vi "Determine XML Dependencies Paths.vi"(10 "Execution Mode":T1, 11 "Targets":enum16{"Linux_x64", "Windows", "All"}(ring)) -> (1 "Targets":string[](array[string]), 2 "Target Paths":string[](array[string]), 3 "Source Paths":string[](array[string]))   [LabVIEW 2026, in "NIVS_CDEW_MetaDataObj.lvclass"]
uses:
  Types/Execution Modes.ctl
  NIVS_CDEW_MetaDataObj.lvclass
  NIVS_CDEW_MetaDataObj.lvclass/NIVS_CDEW_MetaDataObj.ctl
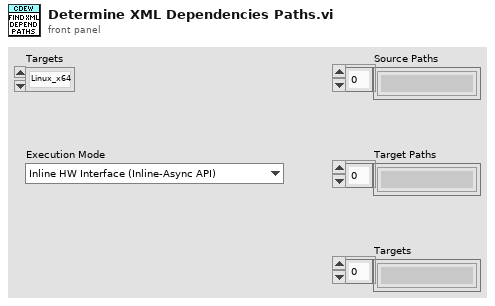
[diagram p1: front panel]
types:
  T1 = typedef "NIVS_CDEW_MetaDataObj.lvclass/Execution Modes.ctl" = enum16{"Inline HW Interface (Inline-Async API)", "Inline HW Interface", "Inline Timing and Sync"}
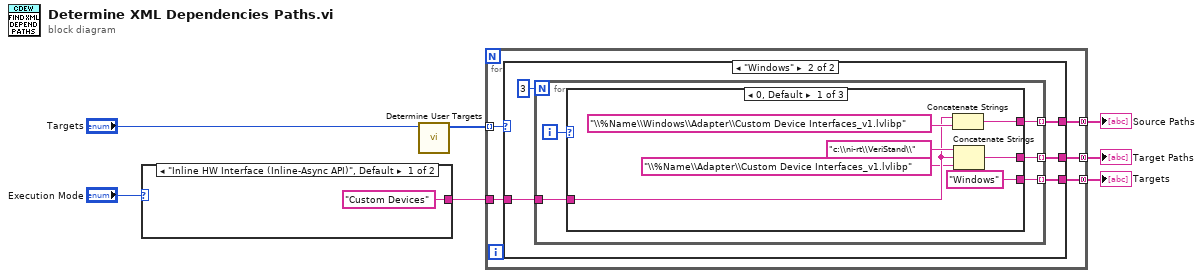
[diagram p0: block diagram]
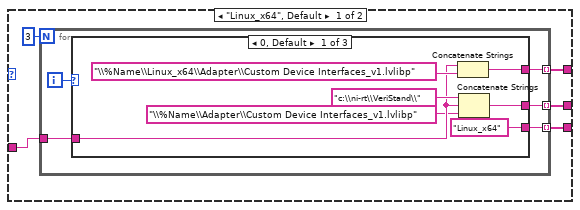
[diagram p2: hidden frame]
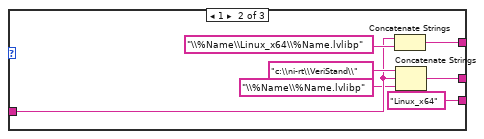
[diagram p3: hidden frame]
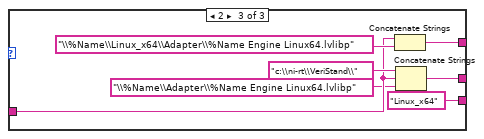
[diagram p4: hidden frame]
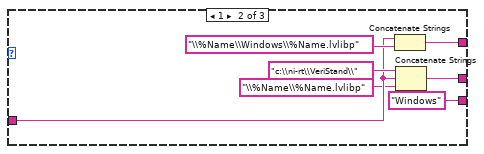
[diagram p5: hidden frame]
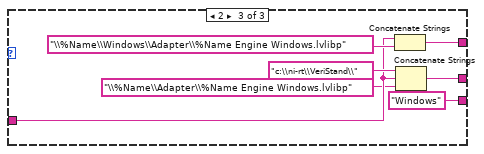
[diagram p6: hidden frame]
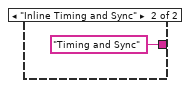
[diagram p7: hidden frame]
diagram:
  n1 = case shown="\"Inline HW Interface (Inline-Async API)\", Default" "Execution Mode" {
    tunnel: ["Custom Devices" "Timing and Sync"] -> w4
    frame "Inline HW Interface (Inline-Async API)", Default {
    }
    frame "Inline Timing and Sync" {
    }
  }
  n2 = call "Determine User Targets.vi"("Targets"="Targets") -> ("User Configured Targets"=w5:enum16{"Linux_x64", "Windows", "All"}[])  [unwired: 10 in]
  n3 = for {
    tunnel: [w14] -> w2 mode=concatenating
    tunnel: [w13] -> w3 mode=concatenating
    tunnel: [w12] -> w1 mode=concatenating
    tunnel: w5 -> [w11] mode=indexing
    tunnel: w4 -> [w10]
    n4 = case shown="\"Windows\"" w11 {
      tunnel: [w19 w50] -> w14
      tunnel: [w18 w49] -> w13
      tunnel: [w17 w48] -> w12
      tunnel: w10 -> [w15 w46]
      frame "Linux_x64", Default {
        n5 = for {
          N: 3 -> [_]
          tunnel: [w24] -> w19 mode=indexing
          tunnel: [w23] -> w18 mode=indexing
          tunnel: [w22] -> w17 mode=indexing
          tunnel: w15 -> [w20]
          i -> [w21]
          n6 = case shown="0, Default" w21 {
            tunnel: [w26 w33 w40] -> w24
            tunnel: [w30 w37 w44] -> w23
            tunnel: ["Linux_x64" ("Tag Data") "Linux_x64" ("Tag Data") "Linux_x64" ("Tag Data")] -> w22
            tunnel: w20 -> [w28 w35 w42]
            frame 0, Default {
              n7 = Concatenate Strings(w28, "\\%Name\\Linux_x64\\Adapter\\Custom Device Interfaces_v1.lvlibp" ("Tag Data")) -> (w30:string)
              n8 = Concatenate Strings("c:\\ni-rt\\VeriStand\\" ("Tag Data"), w28, "\\%Name\\Adapter\\Custom Device Interfaces_v1.lvlibp" ("Tag Data")) -> (w26:string)
            }
            frame 1 {
              n9 = Concatenate Strings(w35, "\\%Name\\Linux_x64\\%Name.lvlibp" ("Tag Data")) -> (w37:string)
              n10 = Concatenate Strings("c:\\ni-rt\\VeriStand\\" ("Tag Data"), w35, "\\%Name\\%Name.lvlibp" ("Tag Data")) -> (w33:string)
            }
            frame 2 {
              n11 = Concatenate Strings(w42, "\\%Name\\Linux_x64\\Adapter\\%Name Engine Linux64.lvlibp" ("Tag Data")) -> (w44:string)
              n12 = Concatenate Strings("c:\\ni-rt\\VeriStand\\" ("Tag Data"), w42, "\\%Name\\Adapter\\%Name Engine Linux64.lvlibp" ("Tag Data")) -> (w40:string)
            }
          }
        }
      }
      frame "Windows" {
        n13 = for {
          N: 3 -> [_]
          tunnel: [w55] -> w50 mode=indexing
          tunnel: [w54] -> w49 mode=indexing
          tunnel: [w53] -> w48 mode=indexing
          tunnel: w46 -> [w51]
          i -> [w52]
          n14 = case shown="0, Default" w52 {
            tunnel: [w57 w64 w71] -> w55
            tunnel: [w61 w68 w75] -> w54
            tunnel: ["Windows" ("Tag Data") "Windows" ("Tag Data") "Windows" ("Tag Data")] -> w53
            tunnel: w51 -> [w59 w66 w73]
            frame 0, Default {
              n15 = Concatenate Strings(w59, "\\%Name\\Windows\\Adapter\\Custom Device Interfaces_v1.lvlibp" ("Tag Data")) -> (w61:string)
              n16 = Concatenate Strings("c:\\ni-rt\\VeriStand\\" ("Tag Data"), w59, "\\%Name\\Adapter\\Custom Device Interfaces_v1.lvlibp" ("Tag Data")) -> (w57:string)
            }
            frame 1 {
              n17 = Concatenate Strings(w66, "\\%Name\\Windows\\%Name.lvlibp" ("Tag Data")) -> (w68:string)
              n18 = Concatenate Strings("c:\\ni-rt\\VeriStand\\" ("Tag Data"), w66, "\\%Name\\%Name.lvlibp" ("Tag Data")) -> (w64:string)
            }
            frame 2 {
              n19 = Concatenate Strings(w73, "\\%Name\\Windows\\Adapter\\%Name Engine Windows.lvlibp" ("Tag Data")) -> (w75:string)
              n20 = Concatenate Strings("c:\\ni-rt\\VeriStand\\" ("Tag Data"), w73, "\\%Name\\Adapter\\%Name Engine Windows.lvlibp" ("Tag Data")) -> (w71:string)
            }
          }
        }
      }
    }
  }
  "Targets" <- w1
  "Source Paths" <- w3
  "Target Paths" <- w2
